vi "Check Empty Letter.vi"(11 "Letter in":string) -> (3 "Letter Out":string)   [LabVIEW 2015]
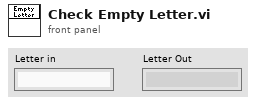
[diagram p1: front panel]
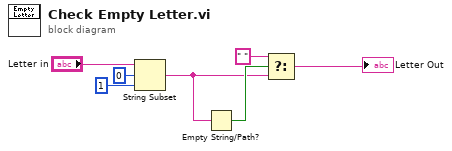
[diagram p0: block diagram]
diagram:
  n1 = String Subset(string="Letter in", offset (0)=0, length (rest)=1 ("length (rest)")) -> (substring=w3:string)
  n2 = Empty String/Path?(string/path=w3) -> (empty?=w7:bool)
  n3 = Select(t=" ", s=w7, f=w3) -> (s? t:f=→"Letter Out":string)
